vi "Test Array.vi"() -> ()   [LabVIEW 2014]
panel:
  out "subarray":i32[](array[numeric])
  out "Array 3":i32[](array[numeric])
  out "Array 2":string[](array[string])
  out "Array":string[][](array[string])
  out "appended array":dbl[][](array[numeric])
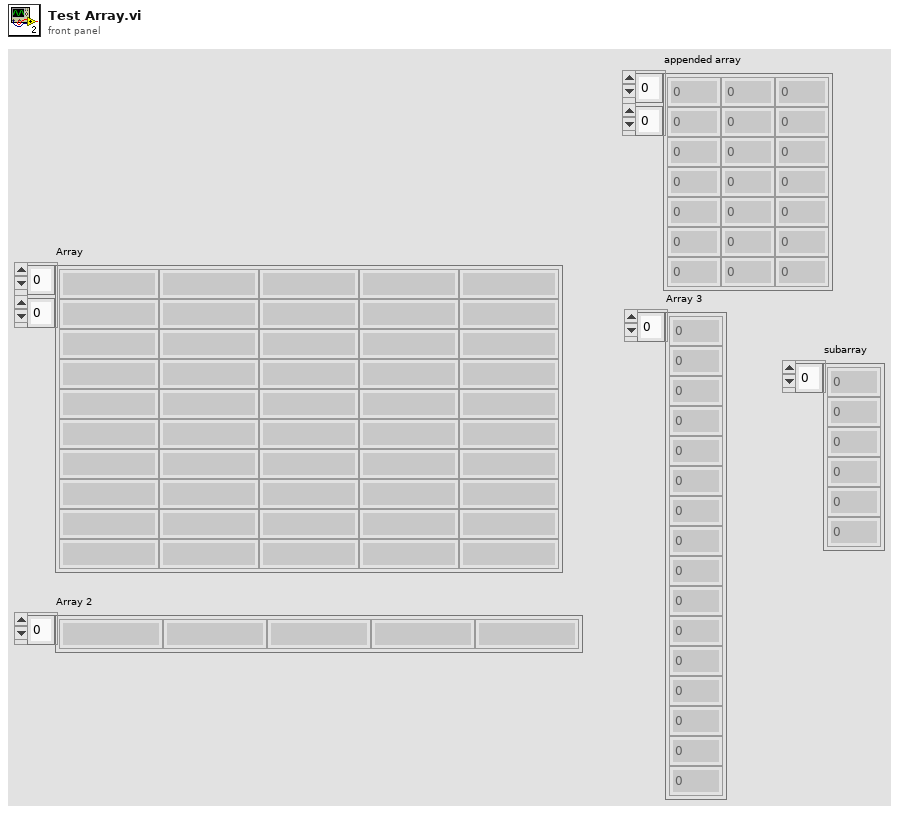
[diagram p1: front panel]
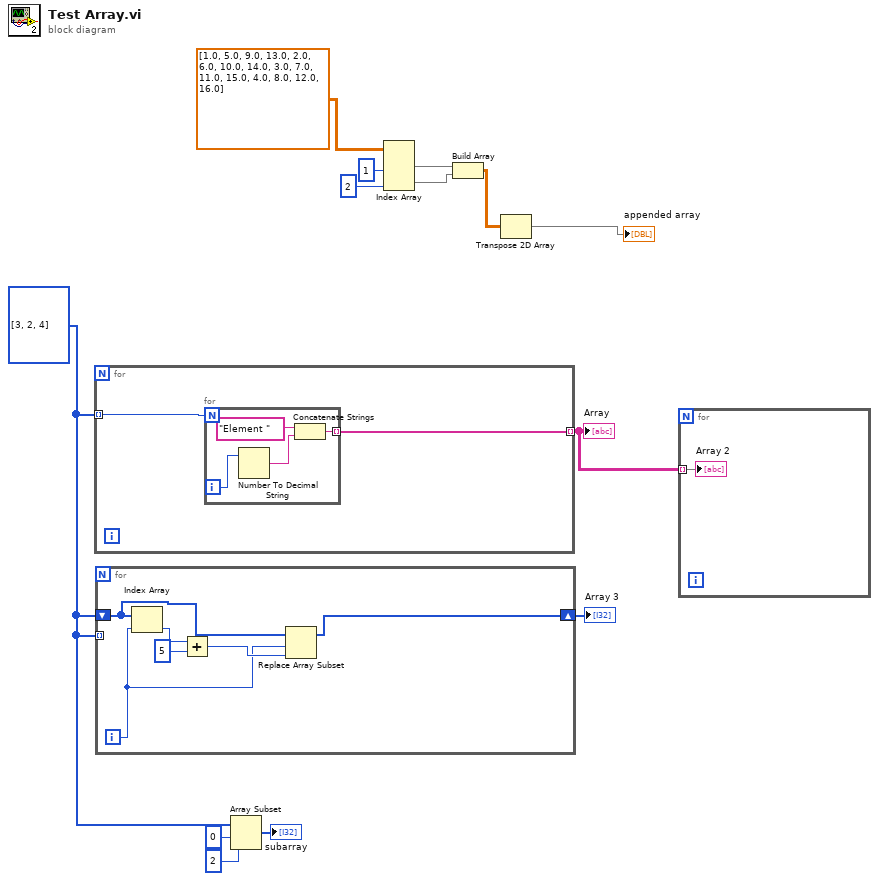
[diagram p0: block diagram]
diagram:
  w4 = i32[] [3, 2, 4]
  n1 = for {
    tunnel: w4 -> [w15] mode=indexing
    tunnel: [w14] -> w6 mode=indexing
    n2 = for {
      N: w15 -> [_]
      tunnel: [w16] -> w14 mode=indexing
      i -> [w17]
      n3 = Number To Decimal String(number=w17) -> (decimal integer string=w18:string)  [unwired: 1 in]
      n4 = Concatenate Strings("Element ", w18) -> (w16:string)
    }
  }
  "Array" <- w6
  n5 = for {
    shift-right: [w20] -> w5
    shift-left: w4 -> [w21]
    tunnel: w4 -> [_] mode=indexing
    i -> [w22]
    n6 = Index Array(array=w21, index=w22) -> (element=w25:i32)
    n7 = Add(x=w25, y=5) -> (x+y=w23:i32)
    n8 = Replace Array Subset(array=w21, new element=w23, index=w22) -> (w20:i32[])
  }
  "Array 3" <- w5
  n9 = Array Subset(array=w4, index=0, length=2) -> (→"subarray":i32[])
  n10 = Index Array(array=dbl[][] [[1.0, 5.0, 9.0, 13.0], [2.0, 6.0, 10.0, 14.0], [3.0, 7.0, 11.0, 15.0], [4.0, 8.0, 12.0, 16.0]], index (col) #1=1 ("disabled index (col)"), index (col) #2=2 ("index (col)")) -> (element #1=w10:dbl[], element #2=w9:dbl[])  [unwired: 2 in]
  n11 = Build Array(w10, w9) -> (w8:dbl[][])
  n12 = Transpose 2D Array(2D array=w8) -> (transposed array=→"appended array":dbl[][])
  n13 = for {
    tunnel: w6 -> [w26] mode=indexing
    "Array 2" <- w26
  }
